vi "Format_RegisterTable.vi"(5 "Register Names":string[](array[string]), 7 "RegMap Data":T1[](array[typedef]) {"Base" format="%.0x"; "Item Count" format="%.0x"; "Value" format="%.0x"; "RegMap"."Mask" format="%.0x"; "Default" format="%.0x"; "Register" format="%.0x"}, 8 "error in (no error)":errorcluster, 11 "Register Data Array":cluster{"String":string, u8}[](array[cluster])) -> (0 "error out":errorcluster, 3 "Register Table":string[][](table))   [LabVIEW 2010]
doc: "This subVI takes register settings data in and updates the register data tables.\n\nInput:\n Register settings - current register settings to update the tables with\n\nOutput:\n Page 0 - Page 0 register data table\n Page 1 - Page 1 register data table"
uses:
  Scan RegMap/TYP_ADSxxxx Register.ctl
  Scan RegMap/TYP_RegMap Item.ctl
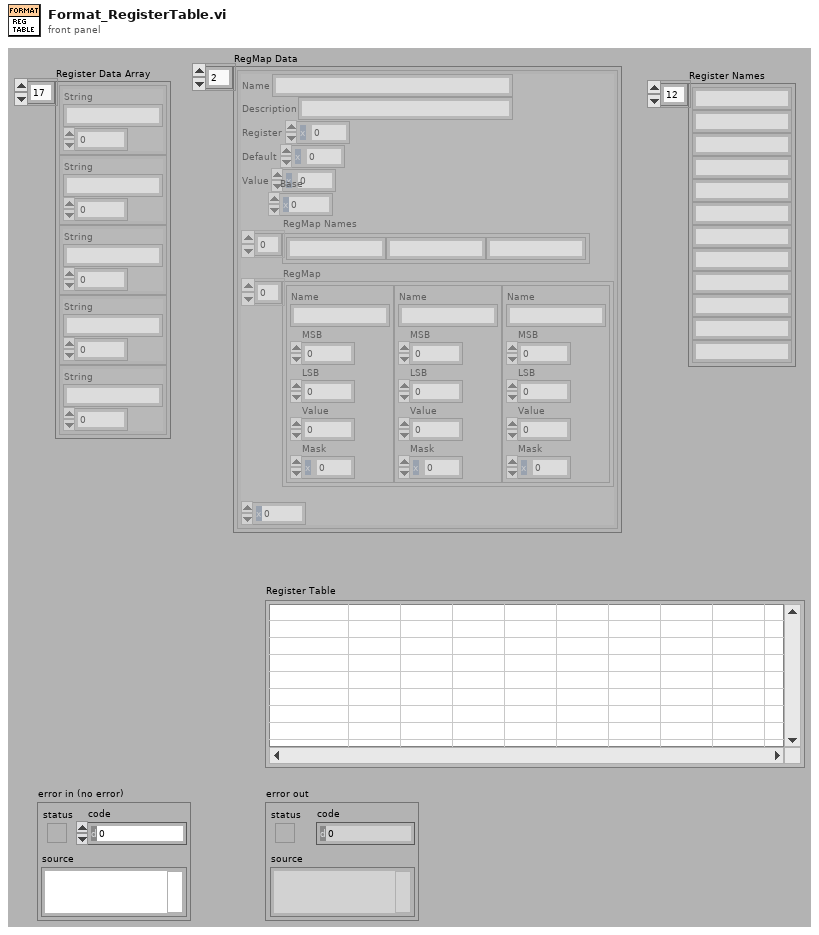
[diagram p1: front panel]
types:
  T1 = typedef "TYP_ADSxxxx Register.ctl" = cluster{"Name":string, "Description":string, "Register":u16, "Default":u16, "Value":u16, "Base":u16, "RegMap Names":string[], "RegMap":T2[], "Item Count":u8}
  T2 = typedef "TYP_RegMap Item.ctl" = cluster{"Name":string, "MSB":u16, "LSB":u16, "Value":u16, "Mask":u16}
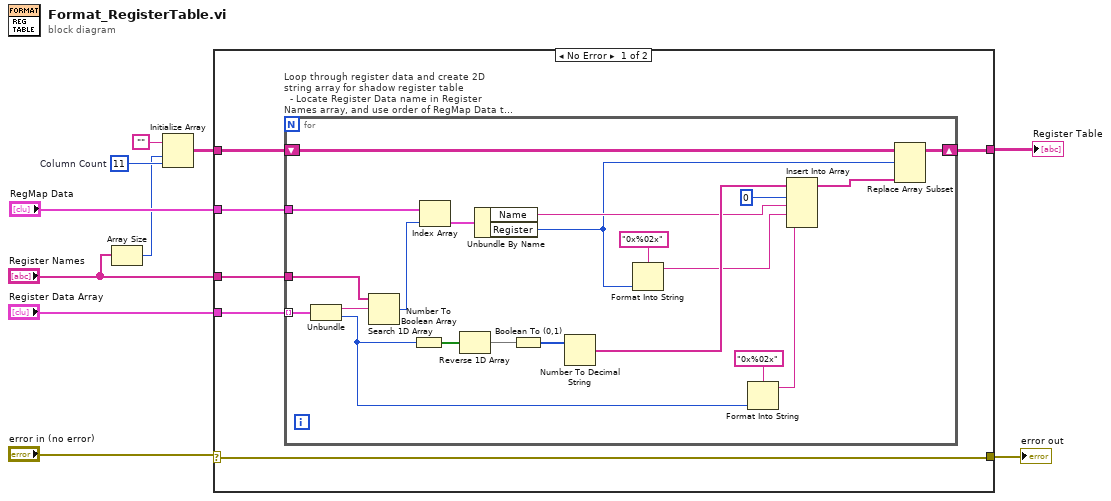
[diagram p0: block diagram]
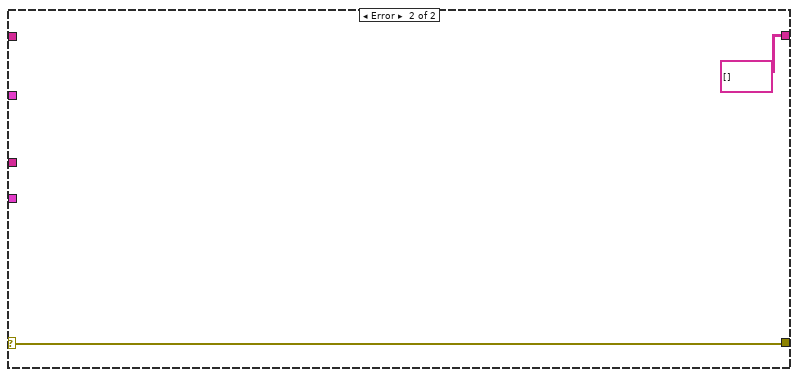
[diagram p2: hidden frame]
diagram:
  w4 = 11  # Column Count
  n1 = Array Size(array="Register Names") -> (size(s)=w1:i32)
  n2 = Initialize Array("", w1, w4) -> (w3:string[][])
  n3 = case shown="No Error" "error in (no error)" {
    selector: "error in (no error)" -> [w13 w39]
    tunnel: "Register Data Array" -> [w16 _]
    tunnel: "Register Names" -> [w15 _]
    tunnel: "RegMap Data" -> [w14 _]
    tunnel: [w11 string[][] []] -> w8
    tunnel: [w13 w39] -> w6
    tunnel: w3 -> [w12 _]
    frame No Error {
      n4 = for "Loop through register data and create 2D string array for shadow register table\n  - Locate Register Data name in Register Names array, and use order of RegMap Data to update item in 2D array." {
        tunnel: w16 -> [w37] mode=indexing
        tunnel: w15 -> [w35]
        tunnel: w14 -> [w34]
        shift-right: [w20] -> w11
        shift-left: w12 -> [w19]
        n5 = Unbundle(w37) -> ("String"=w36:string, w26:u8)
        n6 = Search 1D Array(1D array=w35, element=w36) -> (index of element=w33:i32)  [unwired: 1 out]
        n7 = Number To Boolean Array(number=w26) -> (Boolean array=w28:bool[])
        n8 = Index Array(array=w34, index=w33) -> (element=w32:T1)
        n9 = Reverse 1D Array(array=w28) -> (reversed array=w21:bool[])
        n10 = Unbundle By Name(w32) -> ("Name"=w29:string, "Register"=w17:u16)
        n11 = Boolean To (0,1)(Boolean=w21) -> (0, 1=w27:i16[])
        n12 = Number To Decimal String(number=w27) -> (decimal integer string=w31:string[])  [unwired: 1 out]
        n13 = Format Into String(format string="0x%02x", w17) -> (resulting string=w23:string)  [unwired: 2 in, 1 out]
        n14 = Format Into String(format string="0x%02x", w26) -> (resulting string=w22:string)  [unwired: 2 in, 1 out]
        n15 = Insert Into Array(array=w31, index=0, new element #1=w29, new element #2=w23, new element #3=w22) -> (w18:string[])
        n16 = Replace Array Subset(array=w19, new element=w18, index (row)=w17) -> (w20:string[][])  [unwired: 1 in]
      }
    }
    frame Error {
    }
  }
  "Register Table" <- w8
  "error out" <- w6
